vi "Write Plugins.vi"(8 "error in (no error)":errorcluster, 10 "Plugins":refnum<class "Plugin.lvclass">[](array[class]), 11 "Framework in":refnum<class "Framework.lvclass">) -> (0 "error out":errorcluster, 3 "Framework out":refnum<class "Framework.lvclass">)   [LabVIEW 2016, in "Framework.lvclass"]
uses:
  Framework.lvclass
  Plugin/Plugin.lvclass
  Framework.lvclass/Framework.ctl
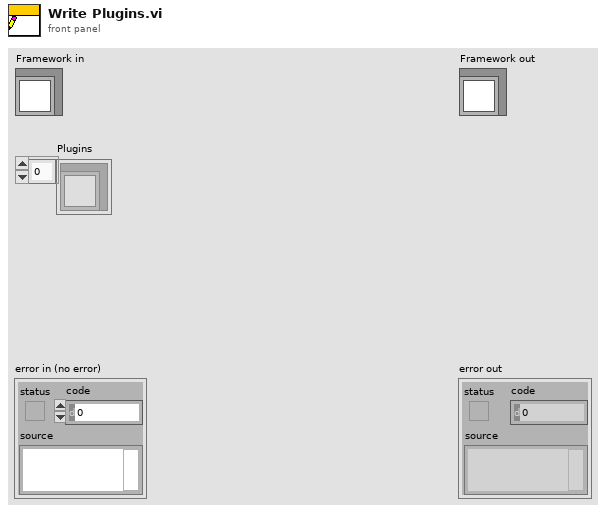
[diagram p1: front panel]
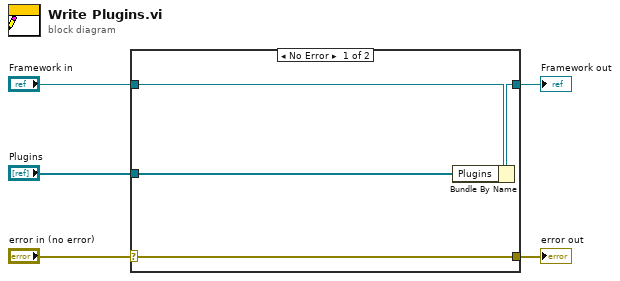
[diagram p0: block diagram]
diagram:
  n1 = case shown="No Error" "error in (no error)" {
    selector: "error in (no error)" -> [w9 w10]
    tunnel: [w9 w10] -> w4
    tunnel: [w7 w11] -> w2
    tunnel: "Framework in" -> [w8 w11]
    tunnel: "Plugins" -> [w6 _]
    frame No Error {
      n2 = Bundle By Name(cluster=w8, "Plugins"=w6) -> (w7:refnum<class "Framework.lvclass">)
    }
    frame Error {
    }
  }
  "error out" <- w4
  "Framework out" <- w2
